vi "listen_for_homing_triggers.vi"(11 "lines":tag) -> ()   [LabVIEW 2021]
uses:
  <vilib>/DAQmx/read.llb/DAQmx Read (Digital Bool 1Line 1Point).vi
  <vilib>/DAQmx/create/channels.llb/DAQmx Create Channel (DI-Digital Input).vi
  <vilib>/DAQmx/miscellaneous.llb/DAQmx Fill In Error Info.vi
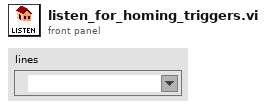
[diagram p1: front panel]
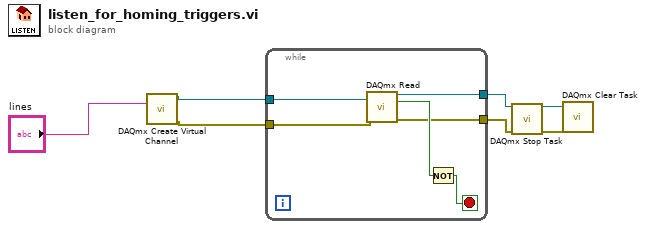
[diagram p0: block diagram]
diagram:
  n1 = call-poly <vilib>:"DAQmx Create Virtual Channel.vi"("lines"="lines") -> ("task out"=w7:refnum<k21>, "error out"=w6:errorcluster)  [unwired: 13 in]
  n2 = while {
    tunnel: w7 -> [w13]
    tunnel: w6 -> [w12]
    tunnel: [w9] -> w5
    tunnel: [w8] -> w4
    stop <- w10 stop-if-true
    n3 = call-poly <vilib>:"DAQmx Read.vi"("task/channels in"=w13, "error in"=w12) -> ("task out"=w9:refnum<k21>, "data"=w11:bool, "error out"=w8:errorcluster)  [unwired: 11 in]
    n4 = Not(x=w11) -> (.not. x?=w10:bool)
  }
  n5 = call <vilib>:"DAQmx Stop Task.vi"("task/channels in"=w5, "error in"=w4) -> ("task out"=w3:refnum<k21>, "error out"=w2:errorcluster)  [unwired: 12 in]
  n6 = call <vilib>:"DAQmx Clear Task.vi"("task in"=w3, "error in"=w2) -> ()  [unwired: 13 in, 1 out]
